vi "DashboardGetvi.vi"(8 "Joystick 2":T1, 9 "Joystick 1":T1) -> ()   [LabVIEW 2018]
uses:
  <vilib>/Rock Robotics/WPI/Joystick/WPI_JoystickDevRef.ctl
  <vilib>/Rock Robotics/WPI/Joystick/WPI_JoystickDeviceEnum.ctl
  <vilib>/Rock Robotics/Network Tables/NT Read Boolean.vi
  <vilib>/Rock Robotics/Network Tables/NT Read Number.vi
  Inputs_DriverStation.vi
  RobotStates.vi
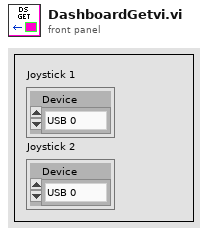
[diagram p1: front panel]
types:
  T1 = typedef "WPI_JoystickDevRef.ctl" = cluster{"Device":T2}
  T2 = typedef "WPI_JoystickDeviceEnum.ctl" = enum16{"USB 0", "USB 1", "USB 2", "USB 3", "USB 4", "USB 5"}
  T3 = cluster{bool, bool, bool, bool, bool, bool, bool, bool, bool, bool, bool, bool, bool, bool}
  T4 = cluster{"Boolean":bool, "Boolean":bool, "Boolean":bool, "Boolean":bool, "Boolean":bool, "Boolean":bool, "Boolean":bool, "Boolean":bool, "Boolean":bool, "Boolean":bool, "Boolean":bool, "Boolean":bool, "Boolean":bool, "Boolean":bool}
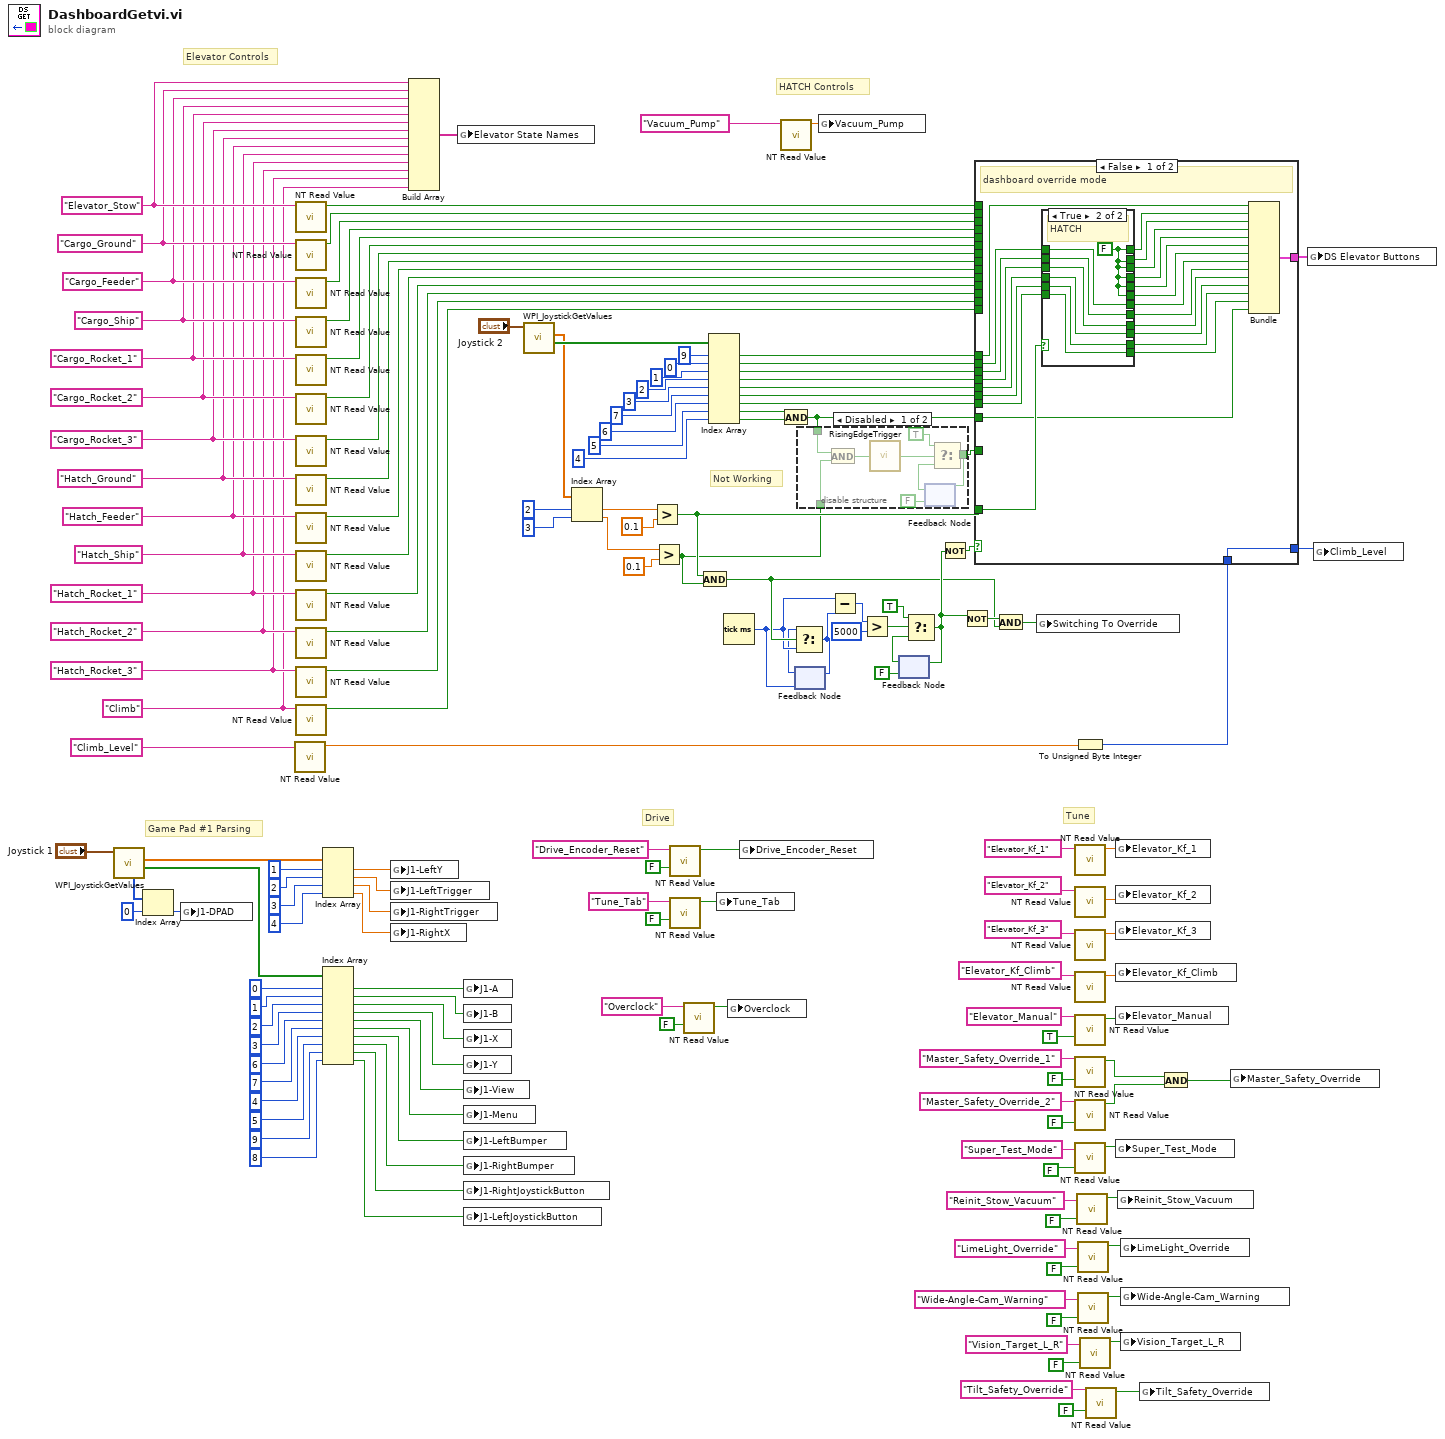
[diagram p0: block diagram]
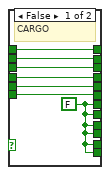
[diagram p3: hidden frame]
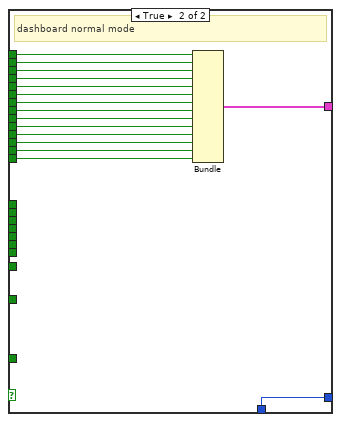
[diagram p4: hidden frame]
diagram:
  w89 = "Climb" ("refnum name")
  w97 = "Hatch_Rocket_3" ("refnum name")
  w98 = "Hatch_Rocket_2" ("refnum name")
  w99 = "Hatch_Rocket_1" ("refnum name")
  w100 = "Hatch_Ship" ("refnum name")
  w101 = "Hatch_Feeder" ("refnum name")
  w102 = "Hatch_Ground" ("refnum name")
  w146 = "Cargo_Rocket_3" ("refnum name")
  w147 = "Cargo_Rocket_2" ("refnum name")
  w148 = "Cargo_Rocket_1" ("refnum name")
  w149 = "Cargo_Ship" ("refnum name")
  w155 = "Cargo_Feeder" ("refnum name")
  w156 = "Cargo_Ground" ("refnum name")
  w157 = "Elevator_Stow" ("refnum name")
  # "Not Working"
  # "Tune"
  # "Drive"
  # "HATCH Controls"
  # "Game Pad #1 Parsing"
  # "Elevator Controls"
  n1 = call <vilib>:"WPI_JoystickGetValues.vi"("JoystickDevRef"="Joystick 1") -> ("Buttons"=w137:bool[], "Axes"=w136:dbl[], "POVs"=w133:i16[])  [unwired: 6 in, 2 out]
  n2 = Index Array(array=w133, index=0) -> (element=w130:i16)
  n3 = global write "Inputs_DriverStation.vi" "J1-DPAD"(w130) -> ()
  n4 = call-poly <vilib>:"NT Read Value.vi"("Name"="Climb_Level" ("refnum name")) -> ("Numeric"=w6:dbl)  [unwired: 9 in, 1 out]
  n5 = call-poly <vilib>:"NT Read Value.vi"("Name"=w157) -> ("Boolean"=w160:bool)  [unwired: 9 in, 1 out]
  n6 = call-poly <vilib>:"NT Read Value.vi"("Name"=w156) -> ("Boolean"=w159:bool)  [unwired: 9 in, 1 out]
  n7 = call-poly <vilib>:"NT Read Value.vi"("Name"=w155) -> ("Boolean"=w158:bool)  [unwired: 9 in, 1 out]
  n8 = call-poly <vilib>:"NT Read Value.vi"("Name"=w149) -> ("Boolean"=w153:bool)  [unwired: 9 in, 1 out]
  n9 = call-poly <vilib>:"NT Read Value.vi"("Name"=w148) -> ("Boolean"=w152:bool)  [unwired: 9 in, 1 out]
  n10 = call-poly <vilib>:"NT Read Value.vi"("Name"=w147) -> ("Boolean"=w151:bool)  [unwired: 9 in, 1 out]
  n11 = call-poly <vilib>:"NT Read Value.vi"("Name"=w146) -> ("Boolean"=w150:bool)  [unwired: 9 in, 1 out]
  n12 = call-poly <vilib>:"NT Read Value.vi"("Name"=w102) -> ("Boolean"=w109:bool)  [unwired: 9 in, 1 out]
  n13 = call-poly <vilib>:"NT Read Value.vi"("Name"=w101) -> ("Boolean"=w108:bool)  [unwired: 9 in, 1 out]
  n14 = call-poly <vilib>:"NT Read Value.vi"("Name"=w100) -> ("Boolean"=w107:bool)  [unwired: 9 in, 1 out]
  n15 = call-poly <vilib>:"NT Read Value.vi"("Name"=w99) -> ("Boolean"=w106:bool)  [unwired: 9 in, 1 out]
  n16 = call-poly <vilib>:"NT Read Value.vi"("Name"=w98) -> ("Boolean"=w105:bool)  [unwired: 9 in, 1 out]
  n17 = call-poly <vilib>:"NT Read Value.vi"("Name"=w97) -> ("Boolean"=w104:bool)  [unwired: 9 in, 1 out]
  n18 = call-poly <vilib>:"NT Read Value.vi"("Name"=w89) -> ("Boolean"=w88:bool)  [unwired: 9 in, 1 out]
  n19 = Index Array(array=w136, index #1=1 ("index"), index #2=2 ("index"), index #3=3 ("index"), index #4=4 ("index")) -> (element #1=w123:dbl, element #2=w124:dbl, element #3=w125:dbl, element #4=w122:dbl)
  n20 = Index Array(array=w137, index #1=0 ("index"), index #2=1 ("index"), index #3=2 ("index"), index #4=3 ("index"), index #5=6 ("index"), index #6=7 ("index"), index #7=4 ("index"), index #8=5 ("index"), index #9=9 ("index"), index #10=8 ("index")) -> (element #1=w129:bool, element #2=w128:bool, element #3=w127:bool, element #4=w126:bool, element #5=w86:bool, element #6=w82:bool, element #7=w79:bool, element #8=w78:bool, element #9=w76:bool, element #10=w71:bool)
  n21 = global write "Inputs_DriverStation.vi" "J1-LeftY"(w123) -> ()
  n22 = global write "Inputs_DriverStation.vi" "J1-LeftTrigger"(w124) -> ()
  n23 = global write "Inputs_DriverStation.vi" "J1-RightTrigger"(w125) -> ()
  n24 = global write "Inputs_DriverStation.vi" "J1-RightX"(w122) -> ()
  n25 = Build Array(w157, w156, w155, w149, w148, w147, w146, w102, w101, w100, w99, w98, w97, w89) -> (w154:string[])
  n26 = global write "RobotStates.vi" "Elevator State Names"(w154) -> ()
  n27 = global write "Inputs_DriverStation.vi" "J1-A"(w129) -> ()
  n28 = global write "Inputs_DriverStation.vi" "J1-B"(w128) -> ()
  n29 = global write "Inputs_DriverStation.vi" "J1-X"(w127) -> ()
  n30 = global write "Inputs_DriverStation.vi" "J1-Y"(w126) -> ()
  n31 = global write "Inputs_DriverStation.vi" "J1-View"(w86) -> ()
  n32 = global write "Inputs_DriverStation.vi" "J1-Menu"(w82) -> ()
  n33 = global write "Inputs_DriverStation.vi" "J1-LeftBumper"(w79) -> ()
  n34 = global write "Inputs_DriverStation.vi" "J1-RightBumper"(w78) -> ()
  n35 = global write "Inputs_DriverStation.vi" "J1-RightJoystickButton"(w76) -> ()
  n36 = global write "Inputs_DriverStation.vi" "J1-LeftJoystickButton"(w71) -> ()
  n37 = call <vilib>:"WPI_JoystickGetValues.vi"("JoystickDevRef"="Joystick 2") -> ("Buttons"=w66:bool[], "Axes"=w50:dbl[])  [unwired: 6 in, 3 out]
  n38 = Index Array(array=w50, index #1=2 ("index"), index #2=3 ("index")) -> (element #1=w49:dbl, element #2=w45:dbl)
  n39 = Greater?(x=w49, y=0.1) -> (0:w44:bool)
  n40 = Greater?(x=w45, y=0.1) -> (0:w32:bool)
  n41 = call-poly <vilib>:"NT Read Value.vi"("Default Value"=FALSE, "Name"="Drive_Encoder_Reset" ("refnum name")) -> ("Boolean"=w110:bool)  [unwired: 8 in, 1 out]
  n42 = call-poly <vilib>:"NT Read Value.vi"("Default Value"=FALSE, "Name"="Tune_Tab" ("refnum name")) -> ("Boolean"=w73:bool)  [unwired: 8 in, 1 out]
  n43 = call-poly <vilib>:"NT Read Value.vi"("Default Value"=FALSE, "Name"="Overclock" ("refnum name")) -> ("Boolean"=w20:bool)  [unwired: 8 in, 1 out]
  n44 = And(x=w44, y=w32) -> (x .and. y?=w26:bool)
  n45 = Index Array(array=w66, index #1=9 ("index"), index #2=0 ("index"), index #3=1 ("index"), index #4=2 ("index"), index #5=3 ("index"), index #6=7 ("index"), index #7=6 ("index"), index #8=5 ("index"), index #9=4 ("index")) -> (element #1=w64:bool, element #2=w62:bool, element #3=w60:bool, element #4=w58:bool, element #5=w56:bool, element #6=w54:bool, element #7=w52:bool, element #8=w35:bool, element #9=w34:bool)
  n46 = global write "Inputs_DriverStation.vi" "Tune_Tab"(w73) -> ()
  n47 = Tick Count (ms)() -> (millisecond timer value=w24:u32)
  n48 = global write "Inputs_DriverStation.vi" "Overclock"(w20) -> ()
  n49 = global write "Inputs_DriverStation.vi" "Drive_Encoder_Reset"(w110) -> ()
  n50 = call-poly <vilib>:"NT Read Value.vi"("Name"="Vacuum_Pump" ("refnum name")) -> ("Numeric"=w113:dbl)  [unwired: 9 in, 1 out]
  n51 = And(x=w35, y=w34) -> (x .and. y?=w33:bool)
  n52 = feedback #1(w24) -> (w23:u32)
  n53 = Select(t=w23, s=w26, f=w24) -> (s? t:f=w30:u32)
  n54 = feedback-in #1(w30) -> ()
  n55 = disable-structure shown="Disabled" {
    disable-tunnel: w33 -> [w168 _]
    disable-tunnel: w32 -> [w167 _]
    disable-tunnel: [w161 _] -> w31
    frame Disabled {
      n56 = And(x=w168, y=w167) -> (x .and. y?=w166:bool)
      n57 = call "RisingEdgeTrigger.vi"("Raw Signal"=w166) -> ("Trigger"=w162:bool)
      n58 = feedback #2(FALSE) -> (w164:bool)
      n59 = Select(t=TRUE, s=w162, f=w164) -> (s? t:f=w161:bool)
      n60 = feedback-in #2(w161) -> ()
    }
    frame Enabled {
    }
  }
  n61 = global write "Inputs_DriverStation.vi" "Vacuum_Pump"(w113) -> ()
  n62 = Subtract(x=w24, y=w30) -> (x-y=w29:u32)
  n63 = Greater?(x=w29, y=u32 5000) -> (0:w42:bool)
  n64 = feedback #3(FALSE) -> (w40:bool)
  n65 = Select(t=TRUE, s=w42, f=w40) -> (s? t:f=w27:bool)
  n66 = feedback-in #3(w27) -> ()
  n67 = Not(x=w27) -> (.not. x?=w38:bool)
  n68 = Not(x=w27) -> (.not. x?=w28:bool)
  n69 = And(x=w28, y=w26) -> (x .and. y?=w25:bool)
  n70 = global write "Inputs_DriverStation.vi" "Switching To Override"(w25) -> ()
  n71 = To Unsigned Byte Integer(number=w6) -> (unsigned 8bit integer=w5:u8)
  n72 = case shown="False" w38 {
    tunnel: w160 -> [_ w221]
    tunnel: w159 -> [_ w220]
    tunnel: w158 -> [_ w219]
    tunnel: w153 -> [_ w218]
    tunnel: w152 -> [_ w217]
    tunnel: w151 -> [_ w216]
    tunnel: w150 -> [_ w215]
    tunnel: w109 -> [_ w214]
    tunnel: w108 -> [_ w213]
    tunnel: w107 -> [_ w212]
    tunnel: w106 -> [_ w211]
    tunnel: w105 -> [_ w210]
    tunnel: w104 -> [_ w209]
    tunnel: [w170 w208] -> w103
    tunnel: w88 -> [_ w207]
    tunnel: w64 -> [w191 _]
    tunnel: w62 -> [w190 _]
    tunnel: w60 -> [w188 _]
    tunnel: w58 -> [w186 _]
    tunnel: w56 -> [w185 _]
    tunnel: w54 -> [w184 _]
    tunnel: w52 -> [w183 _]
    tunnel: w44 -> [w182 _]
    tunnel: w33 -> [w181 _]
    tunnel: [w169 w206] -> w4
    tunnel: w31 -> [_ _]
    tunnel: w5 -> [w169 w206]
    frame False {
      # "dashboard override mode"
      n73 = case shown="True" w182 {
        tunnel: w190 -> [w198 w204]
        tunnel: [w198 w205] -> w189
        tunnel: w188 -> [w197 w203]
        tunnel: [w197 w205] -> w187
        tunnel: w186 -> [w196 w202]
        tunnel: [w196 w205] -> w180
        tunnel: w185 -> [w195 w201]
        tunnel: [w195 w205] -> w179
        tunnel: w184 -> [w194 w200]
        tunnel: [w194 w205] -> w178
        tunnel: w183 -> [w193 w199]
        tunnel: [w193 w205] -> w177
        tunnel: [w192 w204] -> w176
        tunnel: [w192 w203] -> w175
        tunnel: [w192 w202] -> w174
        tunnel: [w192 w201] -> w173
        tunnel: [w192 w200] -> w172
        tunnel: [w192 w199] -> w171
        frame False {
          w192 = FALSE
          # "CARGO"
        }
        frame True {
          w205 = FALSE
          # "HATCH"
        }
      }
      n74 = Bundle(w191, w189, w187, w180, w179, w178, w177, w176, w175, w174, w173, w172, w171, w181) -> (w170:T3)  [unwired: 1 in]
    }
    frame True {
      # "dashboard normal mode"
      n75 = Bundle("Boolean"=w221, "Boolean"=w220, "Boolean"=w219, "Boolean"=w218, "Boolean"=w217, "Boolean"=w216, "Boolean"=w215, "Boolean"=w214, "Boolean"=w213, "Boolean"=w212, "Boolean"=w211, "Boolean"=w210, "Boolean"=w209, "Boolean"=w207) -> (w208:T4)  [unwired: 1 in]
    }
  }
  n76 = call-poly <vilib>:"NT Read Value.vi"("Name"="Elevator_Kf_1" ("refnum name")) -> ("Numeric"=w144:dbl)  [unwired: 9 in, 1 out]
  n77 = call-poly <vilib>:"NT Read Value.vi"("Name"="Elevator_Kf_2" ("refnum name")) -> ("Numeric"=w117:dbl)  [unwired: 9 in, 1 out]
  n78 = call-poly <vilib>:"NT Read Value.vi"("Name"="Elevator_Kf_3" ("refnum name")) -> ("Numeric"=w115:dbl)  [unwired: 9 in, 1 out]
  n79 = call-poly <vilib>:"NT Read Value.vi"("Name"="Elevator_Kf_Climb" ("refnum name")) -> ("Numeric"=w84:dbl)  [unwired: 9 in, 1 out]
  n80 = call-poly <vilib>:"NT Read Value.vi"("Default Value"=TRUE, "Name"="Elevator_Manual" ("refnum name")) -> ("Boolean"=w120:bool)  [unwired: 8 in, 1 out]
  n81 = call-poly <vilib>:"NT Read Value.vi"("Default Value"=FALSE, "Name"="Master_Safety_Override_1" ("refnum name")) -> ("Boolean"=w92:bool)  [unwired: 8 in, 1 out]
  n82 = call-poly <vilib>:"NT Read Value.vi"("Default Value"=FALSE, "Name"="Master_Safety_Override_2" ("refnum name")) -> ("Boolean"=w91:bool)  [unwired: 8 in, 1 out]
  n83 = call-poly <vilib>:"NT Read Value.vi"("Default Value"=FALSE, "Name"="Super_Test_Mode" ("refnum name")) -> ("Boolean"=w69:bool)  [unwired: 8 in, 1 out]
  n84 = call-poly <vilib>:"NT Read Value.vi"("Default Value"=FALSE, "Name"="Reinit_Stow_Vacuum" ("refnum name")) -> ("Boolean"=w18:bool)  [unwired: 8 in, 1 out]
  n85 = call-poly <vilib>:"NT Read Value.vi"("Default Value"=FALSE, "Name"="LimeLight_Override" ("refnum name")) -> ("Boolean"=w15:bool)  [unwired: 8 in, 1 out]
  n86 = call-poly <vilib>:"NT Read Value.vi"("Default Value"=FALSE, "Name"="Wide-Angle-Cam_Warning" ("refnum name")) -> ("Boolean"=w11:bool)  [unwired: 8 in, 1 out]
  n87 = call-poly <vilib>:"NT Read Value.vi"("Default Value"=FALSE, "Name"="Vision_Target_L_R" ("refnum name")) -> ("Boolean"=w8:bool)  [unwired: 8 in, 1 out]
  n88 = call-poly <vilib>:"NT Read Value.vi"("Default Value"=FALSE, "Name"="Tilt_Safety_Override" ("refnum name")) -> ("Boolean"=w1:bool)  [unwired: 8 in, 1 out]
  n89 = global write "Inputs_DriverStation.vi" "Elevator_Kf_1"(w144) -> ()
  n90 = global write "Inputs_DriverStation.vi" "Elevator_Kf_2"(w117) -> ()
  n91 = global write "Inputs_DriverStation.vi" "Elevator_Kf_3"(w115) -> ()
  n92 = global write "Inputs_DriverStation.vi" "Elevator_Kf_Climb"(w84) -> ()
  n93 = global write "Inputs_DriverStation.vi" "Elevator_Manual"(w120) -> ()
  n94 = global write "Inputs_DriverStation.vi" "Super_Test_Mode"(w69) -> ()
  n95 = global write "Inputs_DriverStation.vi" "Reinit_Stow_Vacuum"(w18) -> ()
  n96 = global write "Inputs_DriverStation.vi" "LimeLight_Override"(w15) -> ()
  n97 = global write "Inputs_DriverStation.vi" "Wide-Angle-Cam_Warning"(w11) -> ()
  n98 = global write "Inputs_DriverStation.vi" "Vision_Target_L_R"(w8) -> ()
  n99 = global write "Inputs_DriverStation.vi" "Tilt_Safety_Override"(w1) -> ()
  n100 = And(x=w92, y=w91) -> (x .and. y?=w90:bool)
  n101 = global write "Inputs_DriverStation.vi" "Master_Safety_Override"(w90) -> ()
  n102 = global write "Inputs_DriverStation.vi" "DS Elevator Buttons"(w103) -> ()
  n103 = global write "Inputs_DriverStation.vi" "Climb_Level"(w4) -> ()
